vi "Untitled 4.vi"() -> ()   [LabVIEW 2019]
uses:
  <vilib>/myRIO/Express VI/Onboard Devices/Accelerometer/Accelerometer Express VI.xnode
  <vilib>/myRIO/Instrument Drivers/Onboard Devices/Accelerometer/typedefs/Accelerometer Reference.ctl
  <vilib>/myRIO/Instrument Drivers/Onboard Devices/Accelerometer/Accelerometer.lvlib
  <vilib>/myRIO/Common/Instrument Driver Framework/myRIO v1.0/Accelerometer/typedefs/Accelerometer Channels List.ctl
  <vilib>/myRIO/Common/Instrument Driver Framework/myRIO v1.0/Accelerometer/typedefs/Accelerometer Channels Enum.ctl
  <vilib>/myRIO/Common/Instrument Driver Framework/Utilities/typedefs/myRIO Generic Hardware Reference.ctl
  <vilib>/myRIO/Common/Instrument Driver Framework/Utilities/typedefs/myRIO v1.0 Reference.ctl
  <vilib>/myRIO/Common/Instrument Driver Framework/Utilities/typedefs/Generic FPGA Reference.ctl
  <vilib>/myRIO/Common/Instrument Driver Framework/Utilities/typedefs/Hardware Version Enum.ctl
  <vilib>/myRIO/Instrument Drivers/Onboard Devices/Accelerometer/vis/Read.vi
  <vilib>/myRIO/Instrument Drivers/Onboard Devices/Accelerometer/vis/myRIO Accelerometer Open.xnode
  <vilib>/userDefined/High Color/nirio_resource_hc.ctl
  <vilib>/myRIO/Common/Instrument Driver Framework/myRIO v1.0/Accelerometer/vis/myRIO v1.1 Open Accelerometer.vi
  <vilib>/myRIO/Common/Instrument Driver Framework/Utilities/vis/Is FPGA Ref Available.vi
  <vilib>/myRIO/Express VI/Onboard Devices/Button/Button Express VI.xnode
  <vilib>/myRIO/Instrument Drivers/Onboard IO/DIO/vis/Read.vi
  <vilib>/myRIO/Instrument Drivers/Onboard IO/DIO/DIO.lvlib
  <vilib>/myRIO/Common/Instrument Driver Framework/myRIO v1.0/DIO/typedefs/DIO Channels Enum.ctl
  <vilib>/myRIO/Common/Instrument Driver Framework/myRIO v1.0/DIO/typedefs/DIO Channels List.ctl
  <vilib>/myRIO/Instrument Drivers/Onboard IO/DIO/typedefs/DIO Reference.ctl
  <vilib>/myRIO/Instrument Drivers/Onboard IO/DIO/vis/myRIO DIO Open.xnode
  <vilib>/myRIO/Common/Instrument Driver Framework/myRIO v1.0/DIO/vis/myRIO v1.1 Open DIO.vi
  <vilib>/myRIO/Express VI/Onboard Devices/LED/LED Express VI.xnode
  <vilib>/myRIO/Instrument Drivers/Onboard IO/DIO/vis/Write.vi
  <vilib>/platform/TimedLoop/XDataNode/XDataNode.xnode
  <vilib>/Platform/TimedLoop/XDataNode/nitl_modes.ctl
  <vilib>/Platform/TimedLoop/XDataNode/XDNodeRunTimeDep.lvlib
  <vilib>/Platform/TimedLoop/XDataNode/wakeup.ctl
  <vilib>/Platform/TimedLoop/XDataNode/timing_clust.ctl
panel:
  in  "stop":bool
  out "Angle_mesuré":dbl
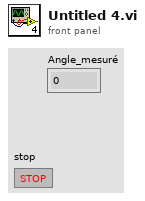
[diagram p1: front panel]
types:
  T1 = typedef "XDNodeRunTimeDep.lvlib/timing_clust.ctl" = cluster{"Expected End [f-1]":u64, "Actual End [f-1]":u64, "Finished Late? [f-1]":bool, "Expected End [i-1]":u64, "Actual End [i-1]":u64, "Finished Late? [i-1]":bool, "Expected Start [i]":u64, "Actual Start [i]":u64, "Expected Start [f]":u64, "Actual Start [f]":u64, "Source Name":string, "Structure Name":string, "Period":i64, "Deadline":i64, "Offset":i64, "Start":i64, "Priority":i32, "Timeout":i32, "Mode":T2, "Wakeup Reason":T3, "Error":errorcluster, "Source Type":string, "Secondary Source Type":string, "Global End Time":u64, "Global Start Time":u64, "Frame Duration":u64, "Iteration Duration":u64, "Assigned CPU":i32, "I/O Scan Engine Mode":u32}
  T2 = typedef "XDNodeRunTimeDep.lvlib/nitl_modes.ctl" = enum32{"No Change", "Process missed periods, maintain original phase", "Discard missed periods, maintain original phase", "Process missed periods, ignore original phase", "Discard missed periods, ignore original phase"}
  T3 = typedef "XDNodeRunTimeDep.lvlib/wakeup.ctl" = enum32{"Normal", "Aborted", "Asynchronous wakeup", "Timing source error", "Timed loop error", "Timeout"}
  T4 = typedef "DIO.lvlib/DIO Reference.ctl" = cluster{"myRIO Reference":T5, "DIO Channels List":T9}
  T5 = typedef "myRIO Generic Hardware Reference.ctl" = cluster{"myRIO Model":T6, "myRIO Hardware Reference":T7}
  T6 = typedef "Hardware Version Enum.ctl" = enum16{"Unknown", "myRIO-1900", "myRIO-1950", "roboRIO", "NI ELVIS RIO CM", "ELVIS III"}
  T7 = typedef "myRIO v1.0 Reference.ctl" = cluster{"Generic FPGA Reference":T8, "Allow multiple opens":bool}
  T8 = typedef "Generic FPGA Reference.ctl" = refnum<k20>
  T9 = typedef "DIO Channels List.ctl" = T10[]
  T10 = typedef "DIO Channels Enum.ctl" = enum16{"Not Connected", "C/DIO0", "C/DIO1", "C/DIO2", "C/DIO3", "C/DIO4", "C/DIO5", "C/DIO6", "C/DIO7", "A/DIO0", "A/DIO1", "A/DIO2", "A/DIO3", "A/DIO4", "A/DIO5", "A/DIO6", "A/DIO7", "A/DIO8", "A/DIO9", "A/DIO10", "A/DIO11", "A/DIO12", "A/DIO13", "A/DIO14", "A/DIO15", "A/DIO16", "A/DIO17", "A/DIO18", "A/DIO19", "B/DIO0", "B/DIO1", "B/DIO2", "B/DIO3", "B/DIO4", "B/DIO5", "B/DIO6", "B/DIO7", "B/DIO8", "B/DIO9", "B/DIO10", "B/DIO11", "B/DIO12", "B/DIO13", "B/DIO14", "B/DIO15", "B/DIO16", "B/DIO17", "B/DIO18", "B/DIO19", "LED0", "LED1", "LED2", "LED3", "Button0", "DIO/DIO0", "DIO/DIO1", "DIO/DIO2", "DIO/DIO3", "DIO/DIO4", "DIO/DIO5", "DIO/DIO6", "DIO/DIO7", "DIO/DIO8", "DIO/DIO9", "SPI/CS0", "SPI/CS1", "SPI/CS2", "SPI/CS3", "LED RADIO (Green)", "LED RADIO (Red)", "LED COMM (Green)", "LED COMM (Red)", "LED MODE (Green)", "LED MODE (Red)"}
  T11 = typedef "nirio_resource_hc.ctl" = tag
  T12 = enum16{"open", "replace", "create", "open or create", "replace or create", "replace or create with confirmation"}
  T13 = typedef "Accelerometer.lvlib/Accelerometer Reference.ctl" = cluster{"myRIO Reference":T5, "Accelerometer Channels List":T14, "LSB Weight":dbl}
  T14 = typedef "Accelerometer Channels List.ctl" = T15[]
  T15 = typedef "Accelerometer Channels Enum.ctl" = enum16{"Not Connected", "X-Axis", "Y-Axis", "Z-Axis"}
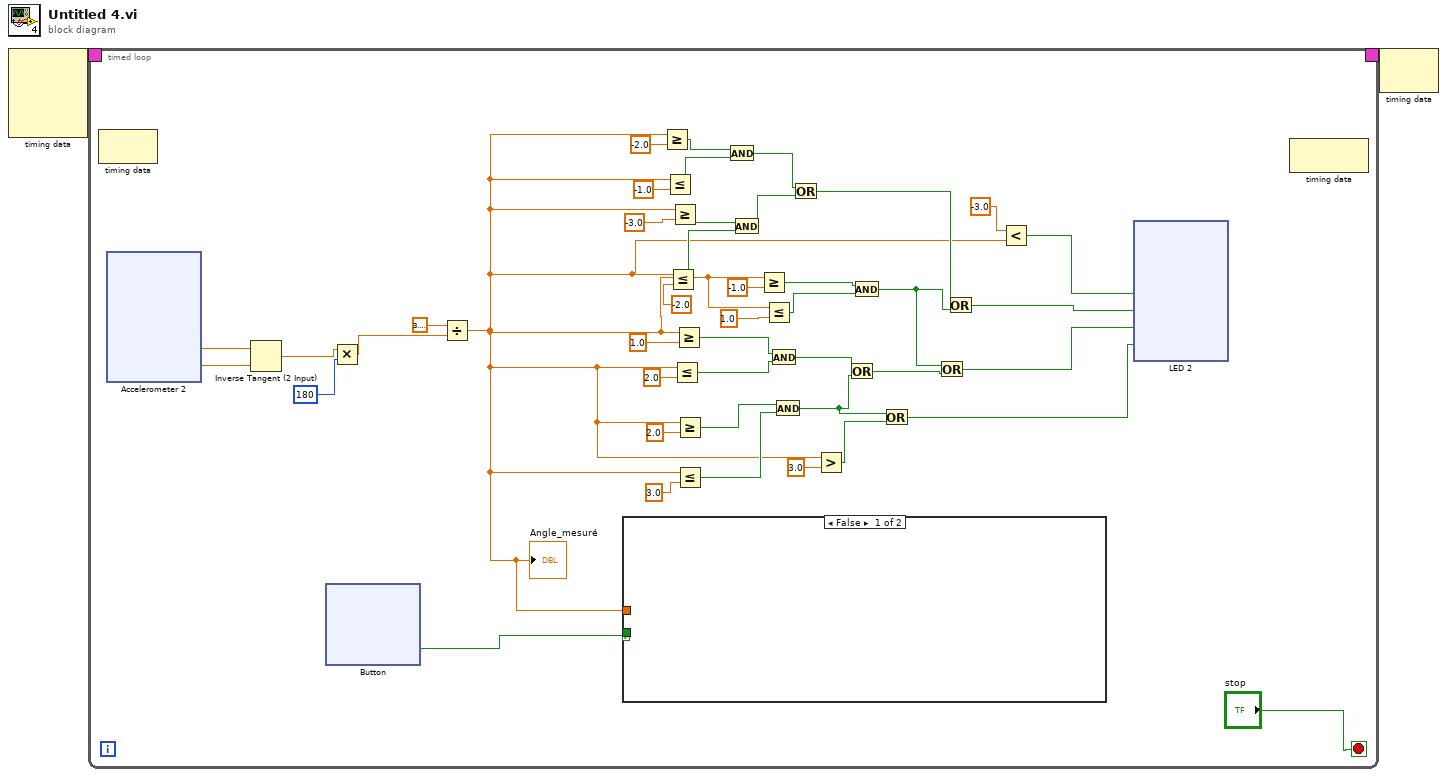
[diagram p0: block diagram]
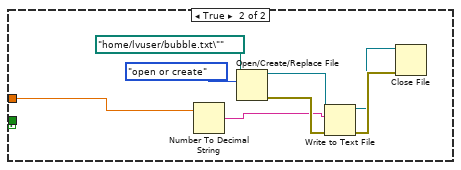
[diagram p2: hidden frame]
diagram:
  n1 = node-c288() -> (w2:T1)  [unwired: 4 in]
  n2 = timed-loop {
    timing: w2 -> [_]
    timing-out: [_] -> w1
    stop <- "stop" stop-if-true
    n3 = node-c288() -> ()  [unwired: 1 in, 1 out]
    n4 = xnode "Accelerometer 2"() -> ("Y-Axis"=w43:dbl, "Z-Axis"=w42:dbl)  [unwired: 1 in, 2 out]
    n5 = Inverse Tangent (2 Input)(1:w42, 2:w43) -> (0:w41:dbl)
    n6 = xnode "Button"() -> ("Value"=w44:bool)  [unwired: 1 in, 1 out]
    n7 = Multiply(x=w41, y=180) -> (x*y=w40:dbl)
    n8 = Divide(x=3.141592653589793, y=w40) -> (x/y=w3:dbl)
    "Angle_mesuré" <- w3
    n9 = case shown="False" w44 {
      selector: w44 -> [_ w120]
      tunnel: [_ w120] -> _
      tunnel: w3 -> [_ w119]
      frame False {
      }
      frame True {
        n10 = Number To Decimal String(number=w119) -> (decimal integer string=w121:string)  [unwired: 1 in]
        n11 = Open/Create/Replace File(file path (use dialog)=path "/home/lvuser/bubble.txt\"", operation (0:open)=T12."open or create") -> (refnum out=w123:refnum<file>, error out=w127:errorcluster)  [unwired: 4 in, 1 out]
        n12 = Write to Text File(file (use dialog)=w123, text=w121, error in=w127) -> (refnum out=w122:refnum<file>, error out=w126:errorcluster)  [unwired: 1 in, 1 out]
        n13 = Close File(refnum=w122, error in=w126) -> ()  [unwired: 2 out]
      }
    }
    n14 = Greater Or Equal?(x=w3, y=-2.0) -> (x >= y?=w30:bool)
    n15 = Less Or Equal?(x=w3, y=-1.0) -> (x <= y?=w29:bool)
    n16 = Less Or Equal?(x=w3, y=-2.0) -> (x <= y?=w27:bool)
    n17 = Greater Or Equal?(x=w3, y=-3.0) -> (x >= y?=w28:bool)
    n18 = Less Or Equal?(x=w3, y=2.0) -> (x <= y?=w21:bool)
    n19 = Greater Or Equal?(x=w3, y=1.0) -> (x >= y?=w22:bool)
    n20 = Greater Or Equal?(x=w3, y=2.0) -> (x >= y?=w20:bool)
    n21 = Less Or Equal?(x=w3, y=3.0) -> (x <= y?=w19:bool)
    n22 = And(x=w30, y=w29) -> (x .and. y?=w26:bool)
    n23 = And(x=w28, y=w27) -> (x .and. y?=w25:bool)
    n24 = Greater Or Equal?(x=w3, y=-1.0) -> (x >= y?=w17:bool)
    n25 = Less Or Equal?(x=w3, y=1.0) -> (x <= y?=w16:bool)
    n26 = And(x=w22, y=w21) -> (x .and. y?=w15:bool)
    n27 = And(x=w20, y=w19) -> (x .and. y?=w13:bool)
    n28 = Or(x=w26, y=w25) -> (x .or. y?=w12:bool)
    n29 = Greater?(x=w3, y=3.0) -> (0:w14:bool)
    n30 = Or(x=w15, y=w13) -> (x .or. y?=w10:bool)
    n31 = And(x=w17, y=w16) -> (x .and. y?=w11:bool)
    n32 = Or(x=w13, y=w14) -> (x .or. y?=w5:bool)
    n33 = Or(x=w11, y=w10) -> (x .or. y?=w6:bool)
    n34 = Or(x=w12, y=w11) -> (x .or. y?=w7:bool)
    n35 = Less?(x=-3.0, y=w3) -> (x < y?=w8:bool)
    n36 = xnode "LED 2"("LED0"=w8, "LED1"=w7, "LED2"=w6, "LED3"=w5) -> ()  [unwired: 1 in, 1 out]
    n37 = node-c288() -> ()  [unwired: 1 in, 1 out]
  }
  n38 = node-c288(w1) -> ()  [unwired: 1 out]
